vi "DS写数据.vi"() -> ()   [LabVIEW 2010]
uses:
  <vilib>/Analysis/NI_AALBase.lvlib
panel:
  out "波形图":dbl[](graph)
  in  "幅值":dbl(slide)=1.0 scale=0.0..10.0
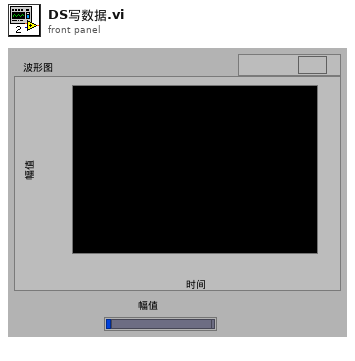
[diagram p1: front panel]
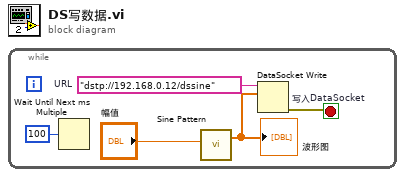
[diagram p0: block diagram]
diagram:
  n1 = while {
    stop <- w2 stop-if-true
    w5 = "dstp://192.168.0.12/dssine"  # URL
    n2 = Wait Until Next ms Multiple(millisecond multiple=u32 100) -> ()  [unwired: 1 out]
    n3 = call <vilib>:"Sine Pattern.vi"("amplitude"="幅值") -> ("Sinusoidal Pattern"=w3:dbl[])  [unwired: 3 in, 1 out]
    "波形图" <- w3
    n4 = DataSocket Write "写入DataSocket"(10:w3, 11:w5) -> (0:w2:errorcluster)  [unwired: 2 in, 2 out]
  }
